vi "Global 1.vi"() -> ()   [LabVIEW 2011]
panel:
  out "Target Info":T1(array[cluster])
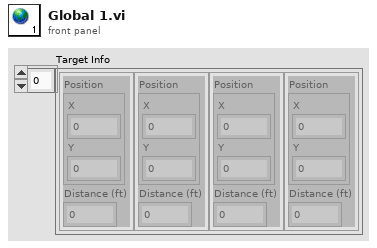
[diagram p1: front panel]
types:
  T1 = cluster{"Position":cluster{"X":dbl, "Y":dbl}, "Distance (ft)":dbl}[]
diagram:
